vi "LCA Is Homing Pos Attained.vi"(8 "error in (no error)":errorcluster caption="Fehler (Eingang, kein Fehler)", 11 "Axis System Handle":i64) -> (0 "error out":errorcluster caption="Fehler (Ausgang)", 3 "Homing Attained":bool)   [LabVIEW 2021, in "labbCAN_MotionControl_API.lvlib"]
doc: "LCA_Func long __stdcall LCA_IsHomingPosAttained(dev_hdl hAxisSystem);"
uses:
  labbCAN_MotionControl_API.lvlib
  labbCAN_MotionControl_API.dll
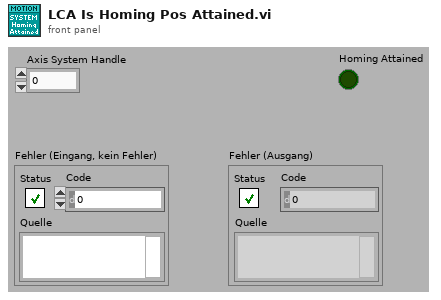
[diagram p1: front panel]
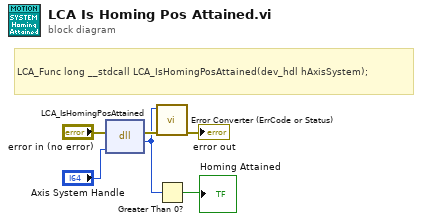
[diagram p0: block diagram]
diagram:
  # "LCA_Func long __stdcall LCA_IsHomingPosAttained(dev_hdl hAxisSystem);"
  n1 = dll-call lib="C:/Users/olaja/AppData/Local/CETONI_SDK/labbCAN_MotionControl_API.*" fn="LCA_IsHomingPosAttained"(error in="error in (no error)", "hAxisSystem"="Axis System Handle") -> (error out=w4:errorcluster, "Rückgabetyp"=w1:i32)  [unwired: 3 in, 1 out]
  n2 = call "Error Converter (ErrCode or Status).vi"("error in (no error)"=w4, "error code"=w1) -> ("error out"=→"error out":errorcluster)  [unwired: 9 in]
  n3 = Greater Than 0?(x=w1) -> (x > 0?=→"Homing Attained":bool)
